vi "Cache_Save PPL Info.vi"(8 "error in":errorcluster, 11 "PPL Details":T1) -> (0 "error out":errorcluster, 1 "Success?":bool, 2 "New Info Loaded?":bool, 3 "Cache Path":path)   [LabVIEW 2020, in "ClassLoader.lvlib"]
uses:
  ClassLoader.lvlib
  Ctl/Ctl_PPL Details.ctl
  <vilib>/Utility/config.llb/Write Key (String).vi
  <vilib>/Utility/config.llb/Write Key (Boolean).vi
  <vilib>/Utility/config.llb/NI_LVConfig.lvlib
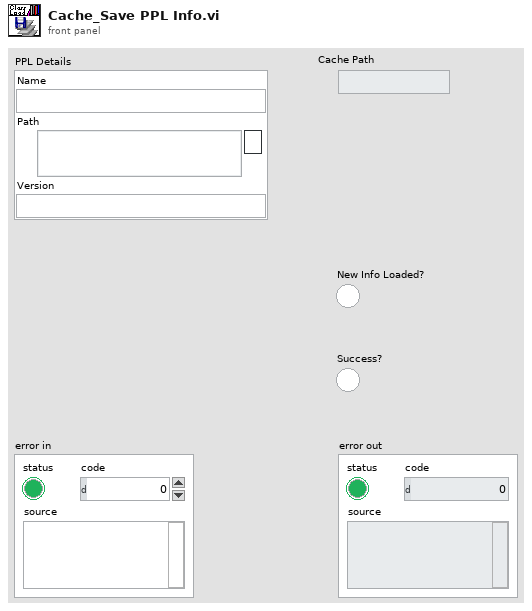
[diagram p1: front panel]
types:
  T1 = typedef "ClassLoader.lvlib/Ctl_PPL Details.ctl" = cluster{"Name":string, "Path":path, "Version":string}
  T2 = typedef "Member VI Info.ctl" = cluster{"qualified name":string, "path":path, "access scope":enum32{"invalid scope", "public", "private", "protected", "community"}, "is dynamic dispatch":bool}
  T3 = typedef "ClassLoader.lvlib/Ctl_Class Info.ctl" = cluster{"Name":string, "Qualified Name":string, "Internal Path":string}
  T4 = cluster{"Is Interface":bool, "Class Info":T3, "Hierarchy Array":T3[], "Member VI info":T2[]}
  T5 = typedef "NI_LVConfig.lvlib/Config Data RefNum.ctl" = refnum<k1>
  T6 = enum32{"invalid scope", "public", "private", "protected", "community"}
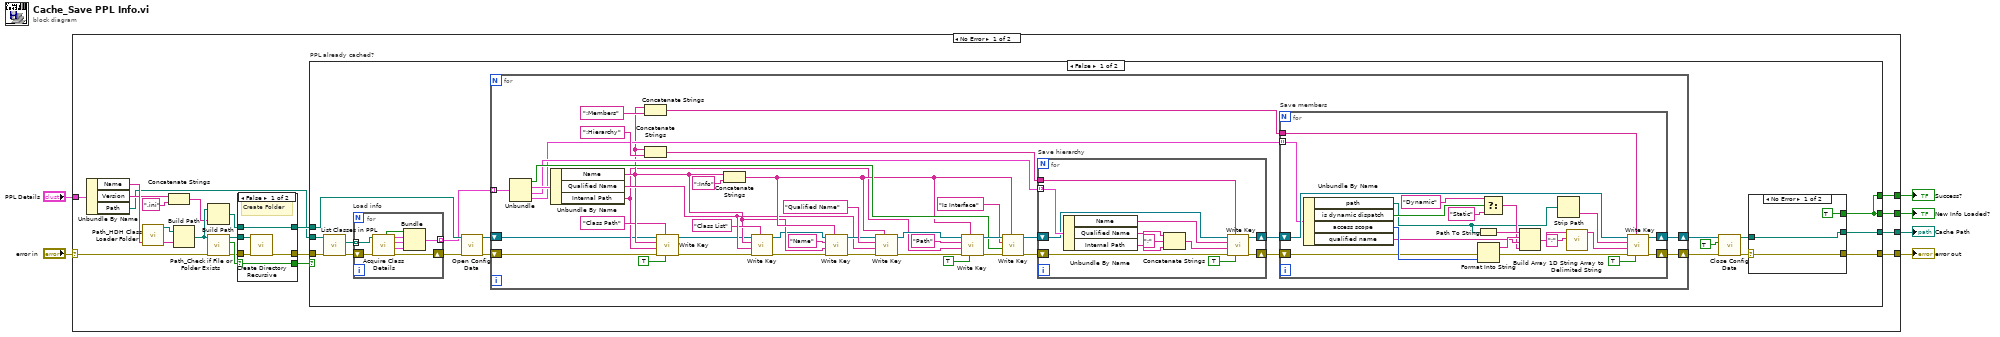
[diagram p0: block diagram]
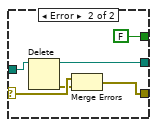
[diagram p2: hidden frame]
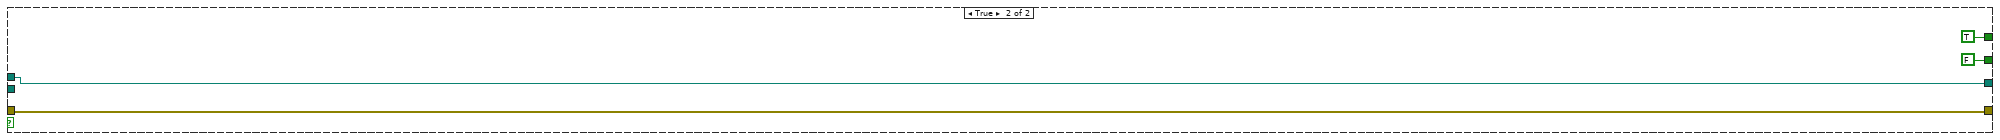
[diagram p3: hidden frame]
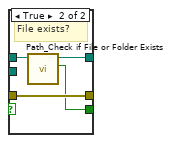
[diagram p4: hidden frame]
diagram:
  n1 = case shown="No Error" "error in" {
    selector: "error in" -> [w20 w146]
    tunnel: [w11 w146] -> w5
    tunnel: "PPL Details" -> [w24 _]
    tunnel: [w13 _] -> w3
    tunnel: [w12 _] -> w2
    tunnel: [w7 _] -> w1
    frame No Error {
      n2 = Unbundle By Name(w24) -> ("Name"=w23:string, "Version"=w18:string, "Path"=w8:path)
      n3 = call "Path_HDH Class Loader Folder.vi"() -> ("HDH\\Class Loader path"=w25:path)  [unwired: 11 in]
      n4 = Concatenate Strings(w18, ".ini" ("string")) -> (w16:string)
      n5 = Build Path(base path=w25, name or relative path=w23) -> (appended path=w19:path)
      n6 = Build Path(base path=w19, name or relative path=w16) -> (appended path=w15:path)
      n7 = call "Path_Check if File or Folder Exists.vi"("File or Folder Path in"=w19) -> ("File or Folder Found?"=w22:bool, "File or Folder Path dub"=w21:path)  [unwired: 9 in]
      n8 = case shown="False" w22 {
        selector: w22 -> [w138 _]
        tunnel: w21 -> [w141 _]
        tunnel: w20 -> [w140 w145]
        tunnel: [w139 w145] -> w10
        tunnel: [w138 w142] -> w14
        tunnel: w15 -> [w137 w144]
        tunnel: [w137 w143] -> w9
        frame False {
          # "Create Folder"
          n9 = call <vilib>:"Create Directory Recursive.vi"("error in (no error)"=w140, "directory"=w141) -> ("error out"=w139:errorcluster)  [unwired: 3 in, 2 out]
        }
        frame True {
          # "File exists?"
          n10 = call "Path_Check if File or Folder Exists.vi"("File or Folder Path in"=w144) -> ("File or Folder Found?"=w142:bool, "File or Folder Path dub"=w143:path)  [unwired: 9 in]
        }
      }
      n11 = case "PPL already cached?" shown="False" w14 {
        tunnel: [w27 FALSE] -> w13
        tunnel: [w27 TRUE] -> w12
        tunnel: [w28 w134] -> w11
        tunnel: w10 -> [w42 w134]
        tunnel: w9 -> [w38 w133]
        tunnel: w8 -> [w41 _]
        tunnel: [w26 w133] -> w7
        frame False {
          n12 = call "List Classes in PPL.vi"("error in"=w42, "PPL Path"=w41) -> ("error out"=w39:errorcluster, "Class Path Array"=w40:path[])  [unwired: 7 in, 1 out]
          n13 = for "Load info" {
            tunnel: w40 -> [w132] mode=indexing
            shift-right: [w130] -> w37
            shift-left: w39 -> [w131]
            tunnel: [w125] -> w31 mode=indexing
            n14 = call "Acquire Class Details.vi"("error in"=w131, "Class Path"=w132) -> ("error out"=w130:errorcluster, "Member VI info"=w126:T2[], "Hierarchy Array"=w127:T3[], "Class Info"=w128:T3, "Is Interface"=w129:bool)  [unwired: 5 in]
            n15 = Bundle("Is Interface"=w129, "Class Info"=w128, "Hierarchy Array"=w127, "Member VI info"=w126) -> (w125:T4)  [unwired: 1 in]
          }
          n16 = call <vilib>:"Open Config Data.vi"("error in (no error)"=w37, "configuration file path"=w38) -> ("error out"=w35:errorcluster, "refnum"=w36:T5)  [unwired: 7 in, 1 out]
          n17 = for {
            shift-right: [w54] -> w34
            shift-left: w36 -> [w53]
            shift-right: [w56] -> w33
            shift-left: w35 -> [w59]
            tunnel: w31 -> [w91] mode=indexing
            n18 = Unbundle(w91) -> ("Is Interface"=w78:bool, "Class Info"=w89:T3, "Hierarchy Array"=w76:T3[], "Member VI info"=w69:T2[])
            n19 = Unbundle By Name(w89) -> ("Name"=w63:string, "Qualified Name"=w65:string, "Internal Path"=w61:string)
            n20 = Concatenate Strings(w63, ":Members" ("key")) -> (w68:string)
            n21 = Concatenate Strings(w63, ":Hierarchy" ("key")) -> (w67:string)
            n22 = call-poly <vilib>:"Write Key.vi"("write raw string? (F)"=TRUE, "section"="Class Path", "error in (no error)"=w59, "value"=w61, "key"=w63, "refnum"=w53) -> ("error out"=w58:errorcluster, "refnum out"=w55:T5)  [unwired: 3 in, 1 out]
            n23 = Concatenate Strings(w63, ":Info" ("section")) -> (w66:string)
            n24 = call-poly <vilib>:"Write Key.vi"("section"="Class List", "error in (no error)"=w58, "value"=w65, "key"=w63, "refnum"=w55) -> ("error out"=w57:errorcluster, "refnum out"=w52:T5)  [unwired: 4 in, 1 out]
            n25 = call-poly <vilib>:"Write Key.vi"("section"=w66, "error in (no error)"=w57, "value"=w63, "key"="Name", "refnum"=w52) -> ("error out"=w88:errorcluster, "refnum out"=w86:T5)  [unwired: 4 in, 1 out]
            n26 = call-poly <vilib>:"Write Key.vi"("section"=w66, "error in (no error)"=w88, "value"=w65, "key"="Qualified Name", "refnum"=w86) -> ("error out"=w83:errorcluster, "refnum out"=w85:T5)  [unwired: 4 in, 1 out]
            n27 = call-poly <vilib>:"Write Key.vi"("write raw string? (F)"=TRUE, "section"=w66, "error in (no error)"=w83, "value"=w61, "key"="Path", "refnum"=w85) -> ("error out"=w77:errorcluster, "refnum out"=w80:T5)  [unwired: 3 in, 1 out]
            n28 = call-poly <vilib>:"Write Key.vi"("section"=w66, "error in (no error)"=w77, "value"=w78, "key"="Is Interface", "refnum"=w80) -> ("error out"=w73:errorcluster, "refnum out"=w75:T5)  [unwired: 4 in, 1 out]
            n29 = for "Save hierarchy" {
              tunnel: w76 -> [w124] mode=indexing
              shift-right: [w116] -> w71
              shift-left: w75 -> [w117]
              tunnel: w67 -> [w123]
              shift-right: [w113] -> w70
              shift-left: w73 -> [w115]
              n30 = Unbundle By Name(w124) -> ("Name"=w122:string, "Qualified Name"=w121:string, "Internal Path"=w119:string)
              n31 = Concatenate Strings(w121, ";" ("string"), w119) -> (w118:string)
              n32 = call-poly <vilib>:"Write Key.vi"("write raw string? (F)"=TRUE, "section"=w123, "error in (no error)"=w115, "value"=w118, "key"=w122, "refnum"=w117) -> ("error out"=w113:errorcluster, "refnum out"=w116:T5)  [unwired: 3 in, 1 out]
            }
            n33 = for "Save members" {
              tunnel: w69 -> [w107] mode=indexing
              shift-right: [w110] -> w54
              shift-left: w71 -> [w111]
              tunnel: w68 -> [w112]
              shift-right: [w108] -> w56
              shift-left: w70 -> [w100]
              n34 = Unbundle By Name(w107) -> ("path"=w96:path, "is dynamic dispatch"=w105:bool, "access scope"=w101:T6, "qualified name"=w97:string)
              n35 = Path To String(path=w96) -> (string=w95:string)
              n36 = Format Into String(error in=w100, w101) -> (resulting string=w98:string, error out=w99:errorcluster)  [unwired: 2 in]
              n37 = Select(t="Dynamic" ("string"), s=w105, f="Static" ("string")) -> (s? t:f=w102:string)
              n38 = Build Array(w102, w98, w97, w95) -> (w94:string[])
              n39 = Strip Path(path=w96) -> (name=w106:string)  [unwired: 1 out]
              n40 = call <vilib>:"1D String Array to Delimited String.vi"("delimiter"=";" ("string"), "string array"=w94) -> ("delimited string"=w92:string)  [unwired: 9 in]
              n41 = call-poly <vilib>:"Write Key.vi"("write raw string? (F)"=TRUE, "section"=w112, "error in (no error)"=w99, "value"=w92, "key"=w106, "refnum"=w111) -> ("error out"=w108:errorcluster, "refnum out"=w110:T5)  [unwired: 3 in, 1 out]
            }
          }
          n42 = call <vilib>:"Close Config Data.vi"("error in (no error)"=w33, "write file if changed (T)"=TRUE, "refnum"=w34) -> ("error out"=w29:errorcluster, "file path"=w30:path)  [unwired: 7 in]
          n43 = case shown="No Error" w29 {
            selector: w29 -> [w45 w50]
            tunnel: w30 -> [w43 w51]
            tunnel: [w45 w48] -> w28
            tunnel: [TRUE FALSE] -> w27
            tunnel: [w43 w46] -> w26
            frame No Error {
            }
            frame Error {
              n44 = Delete(path (use dialog)=w51) -> (deleted path=w46:path, error out=w49:errorcluster)  [unwired: 4 in, 1 out]
              n45 = Merge Errors(w50, w49) -> (w48:errorcluster)
            }
          }
        }
        frame True {
        }
      }
    }
    frame Error {
    }
  }
  "New Info Loaded?" <- w3
  "error out" <- w5
  "Success?" <- w2
  "Cache Path" <- w1
